vi "Servo Pulse Gen..vi"() -> ()   [LabVIEW 2015]
uses:
  Slide Servo.ctl
  Galobal variable_TI.vi
  Project Setup/Globle Variable/GR_Servo.vi
panel:
  out "Enum":T1
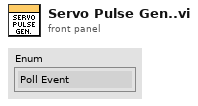
[diagram p1: front panel]
types:
  T1 = typedef "Slide Servo.ctl" = enum16{"Poll Event", "Servo CMD", "Slide Servo Home ", "Exit"}
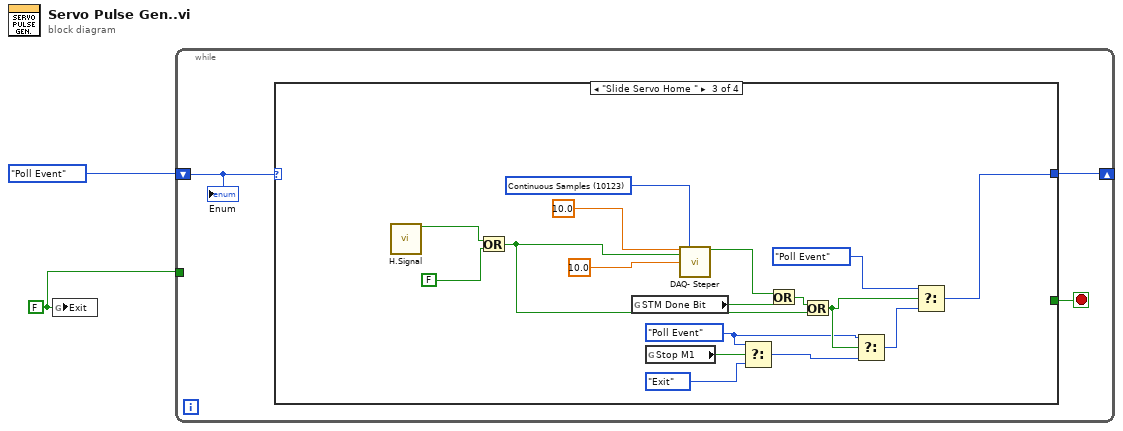
[diagram p0: block diagram]
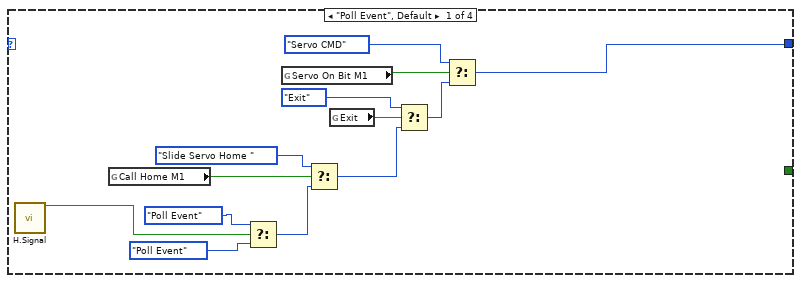
[diagram p2: hidden frame]
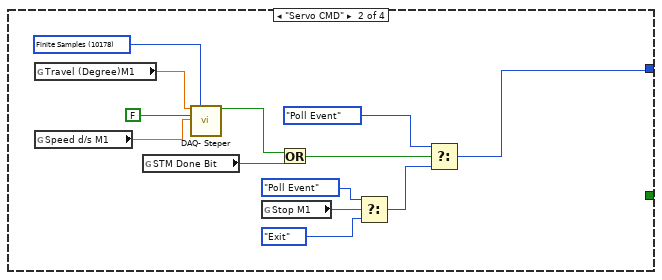
[diagram p3: hidden frame]
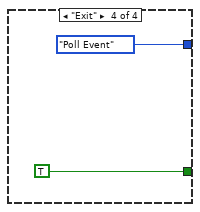
[diagram p4: hidden frame]
diagram:
  w1 = FALSE ("Exit")
  n1 = global write "Galobal variable_TI.vi" "Exit"(w1) -> ()
  n2 = while {
    shift-right: [w4] -> _
    shift-left: Slide_Servo."Poll Event" ("Enum") -> [w5]
    tunnel: w1 -> [_]
    stop <- w3 stop-if-true
    n3 = case shown="\"Slide Servo Home \"" w5 {
      tunnel: [w13 w25 w35 Slide_Servo."Poll Event" ("Enum")] -> w4
      tunnel: [_ _ _ TRUE] -> w3
      frame "Poll Event", Default {
        n4 = call "H.Signal.vi"() -> ("Slide servo home RS"=w9:bool)  [unwired: 11 in, 4 out]
        n5 = global read "Galobal variable_TI.vi" "Call Home M1"() -> (w11:bool)
        n6 = Select(t=Slide_Servo."Poll Event" ("Enum"), s=w9, f=Slide_Servo."Poll Event" ("Enum")) -> (s? t:f=w7:T1)
        n7 = global read "GR_Servo.vi" "Servo On Bit M1"() -> (w16:bool)
        n8 = Select(t=Slide_Servo."Slide Servo Home " ("Enum"), s=w11, f=w7) -> (s? t:f=w10:T1)
        n9 = global read "Galobal variable_TI.vi" "Exit"() -> (w17:bool)
        n10 = Select(t=Slide_Servo."Exit" ("Enum"), s=w17, f=w10) -> (s? t:f=w18:T1)
        n11 = Select(t=Slide_Servo."Servo CMD" ("Enum"), s=w16, f=w18) -> (s? t:f=w13:T1)
      }
      frame "Servo CMD" {
        w19 = 10178 items=["Finite Samples"=10178, "Continuous Samples"=10123, "Hardware Timed Single Point"=12522] ("Mode")
        n12 = global read "GR_Servo.vi" "Travel (Degree)M1"() -> (w30:dbl)
        n13 = global read "GR_Servo.vi" "Speed d/s M1"() -> (w31:dbl)
        n14 = global read "Galobal variable_TI.vi" "STM Done Bit"() -> (w28:bool)
        n15 = call "DAQ- Steper.vi"("Travel (Degree)"=w30, "Mode"=w19, "Home Condition"=FALSE, "Speed d/s"=w31) -> ("Task Done Bit"=w29:bool)  [unwired: 10 in, 1 out]
        n16 = global read "Galobal variable_TI.vi" "Stop M1"() -> (w24:bool)
        n17 = Or(x=w29, y=w28) -> (x .or. y?=w27:bool)
        n18 = Select(t=Slide_Servo."Poll Event" ("Enum"), s=w24, f=Slide_Servo."Exit" ("Enum")) -> (s? t:f=w21:T1)
        n19 = Select(t=Slide_Servo."Poll Event" ("Enum"), s=w27, f=w21) -> (s? t:f=w25:T1)
      }
      frame "Slide Servo Home " {
        w34 = 10123 items=["Finite Samples"=10178, "Continuous Samples"=10123, "Hardware Timed Single Point"=12522] ("Mode")
        w37 = Slide_Servo."Poll Event" ("Enum")
        n20 = call "H.Signal.vi"() -> ("Slide servo home RS"=w48:bool)  [unwired: 11 in, 4 out]
        n21 = Or(x=w48, y=FALSE) -> (x .or. y?=w42:bool)
        n22 = global read "Galobal variable_TI.vi" "STM Done Bit"() -> (w46:bool)
        n23 = global read "Galobal variable_TI.vi" "Stop M1"() -> (w41:bool)
        n24 = call "DAQ- Steper.vi"("Travel (Degree)"=10.0, "Mode"=w34, "Home Condition"=w42, "Speed d/s"=10.0) -> ("Task Done Bit"=w47:bool)  [unwired: 10 in, 1 out]
        n25 = Select(t=w37, s=w41, f=Slide_Servo."Exit" ("Enum")) -> (s? t:f=w38:T1)
        n26 = Or(x=w47, y=w46) -> (x .or. y?=w43:bool)
        n27 = Or(x=w43, y=w42) -> (x .or. y?=w39:bool)
        n28 = Select(t=w37, s=w39, f=w38) -> (s? t:f=w36:T1)
        n29 = Select(t=Slide_Servo."Poll Event" ("Enum"), s=w39, f=w36) -> (s? t:f=w35:T1)
      }
      frame "Exit" {
      }
    }
    "Enum" <- w5
  }
